vi "Get Dwell Time.vi"(8 "error in (no error)":errorcluster, 11 "VISA resource name":refnum<visa-resource-name>) -> (0 "error out":errorcluster, 1 "output":dbl[unit], 3 "VISA resource name out":refnum<visa-resource-name>)   [LabVIEW 2015, in "SR400.lvlib"]
uses:
  SR400.lvlib
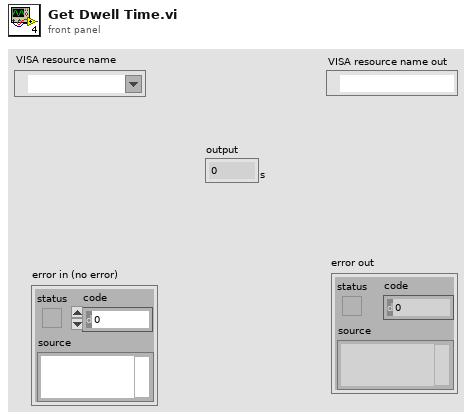
[diagram p1: front panel]
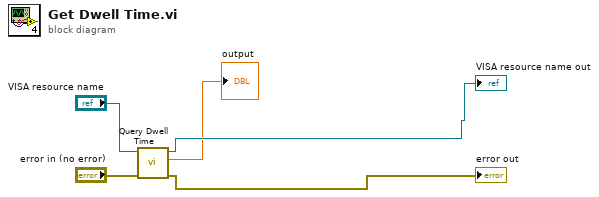
[diagram p0: block diagram]
diagram:
  n1 = call "Query Dwell Time.vi"("error in (no error)"="error in (no error)", "VISA resource name"="VISA resource name") -> ("error out"=→"error out":errorcluster, "output"=→"output":dbl[unit], "VISA resource name out"=→"VISA resource name out":refnum<visa-resource-name>)  [unwired: 7 in]
